vi "OR flags U32.vi"(11 "flags":u32[](array[numeric])) -> (3 "OR'ed flags":u32)   [LabVIEW 2016, in "Linux RT IPC.C.lvlib"]
uses:
  Linux RT IPC.C.lvlib
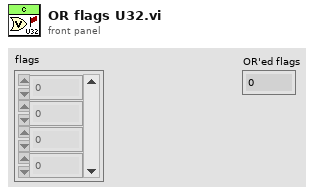
[diagram p1: front panel]
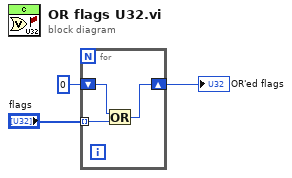
[diagram p0: block diagram]
diagram:
  n1 = for {
    tunnel: "flags" -> [w4] mode=indexing
    shift-right: [w6] -> w1
    shift-left: u32 0 -> [w5]
    n2 = Or(x=w5, y=w4) -> (x .or. y?=w6:u32)
  }
  "OR'ed flags" <- w1
